vi "Create Report Session.vi"(0 "Session Handle in":T3, 7 "Execution":T2, 11 "error in (no error)":errorcluster) -> (4 "Session Handle out":T3, 8 "Report":T1, 15 "error out":errorcluster)   [LabVIEW 2020, in "TSS.lvlib" / "Engine.lvclass"]
uses:
  Engine.lvclass
  Typedefs/Session Handle.ctl
  Execution/Typedefs/Session Handle.ctl
  Execution/Execution.lvclass
  Report/Typedefs/Session Handle.ctl
  Report/Report.lvclass
  Create Report Event Data.ctl
  Engine.lvclass/Engine.ctl
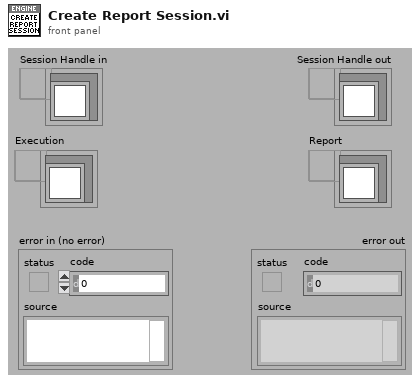
[diagram p1: front panel]
types:
  T1 = typedef "TSS.lvlib/Report.lvclass/Session Handle.ctl" = refnum<data-value>
  T2 = typedef "TSS.lvlib/Execution.lvclass/Session Handle.ctl" = refnum<data-value>
  T3 = typedef "TSS.lvlib/Engine.lvclass/Session Handle.ctl" = refnum<data-value>
  T4 = typedef "TSS.lvlib/Engine.lvclass/Create Report Event Data.ctl" = cluster{"Execution":T2, "Report Notifier":refnum<notifier>}
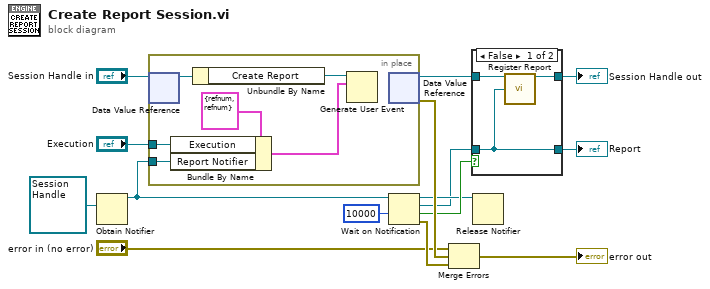
[diagram p0: block diagram]
diagram:
  n1 = Obtain Notifier(notification data type=T1 refnum ("Report")) -> (notifier out=w10:refnum<notifier>)  [unwired: 3 in, 2 out]
  n2 = in-place {
    in-place-border: "Execution" -> [w19]
    in-place-border: w10 -> [w18]
    n3 = in-place-dvr #1("Session Handle in") -> (w21:refnum<class "Engine.lvclass">)  [unwired: 1 out]
    n4 = Bundle By Name(cluster=T4 {"Execution"=refnum, "Report Notifier"=refnum} ("Create Report Event Data"), "Execution"=w19, "Report Notifier"=w18) -> (w16:T4)
    n5 = Unbundle By Name(w21) -> ("Create Report"=w17:refnum<user-event>)
    n6 = Generate User Event(user event=w17, event data cluster=w16) -> ()  [unwired: 2 in, 2 out]
    n7 = in-place-dvr #1() -> (w2:T3, w15:errorcluster)  [unwired: 1 in]
  }
  n8 = Wait on Notification(notifier=w10, timeout in ms (-1)=10000) -> (notifier out=w6:refnum<notifier>, notification=w5:T1, timed out?=w8:bool, error out=w14:errorcluster)  [unwired: 2 in]
  n9 = Merge Errors("error in (no error)", w15, w14) -> (→"error out":errorcluster)
  n10 = case shown="False" w8 {
    tunnel: w5 -> [w23 _]
    tunnel: [w23 _] -> w7
    tunnel: w2 -> [w24 w25]
    tunnel: [w22 w25] -> w1
    frame False {
      n11 = call "Register Report.vi"("Engine  In"=w24, "Report"=w23) -> ("Engine"=w22:T3)  [unwired: 12 in, 1 out]
    }
    frame True {
    }
  }
  "Session Handle out" <- w1
  "Report" <- w7
  n12 = Release Notifier(notifier=w6) -> ()  [unwired: 2 in, 3 out]
